vi "MTM2_logEvent_logLevel.vi"(8 "error in (no error)":errorcluster, 11 "logevent_logLevel_Ctl":T1) -> (0 "error out":errorcluster, 2 "function return":i32, 3 "logevent_logLevel_Ctl out":T1)   [LabVIEW 2018, in "SALLV_MTM2.lvlib"]
doc: "int MTM2_shm_logEvent_logLevelLV(MTM2_logevent_logLevelLV *logevent_logLevel_Ctl );"
uses:
  SALLV_MTM2.lvlib
  DataTypes/logevent_logLevel.ctl
  SALLV_MTM2.so
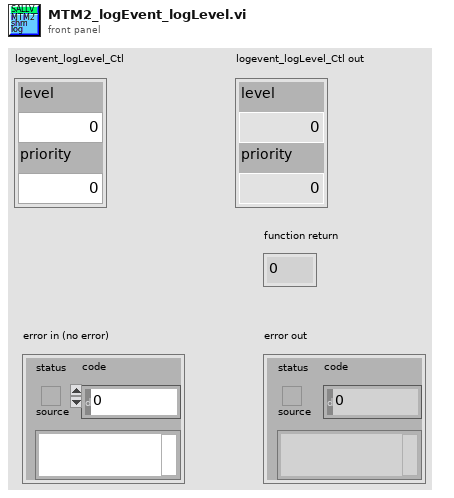
[diagram p1: front panel]
types:
  T1 = typedef "SALLV_MTM2.lvlib/logevent_logLevel.ctl" = cluster{"level":i32, "priority":i32}
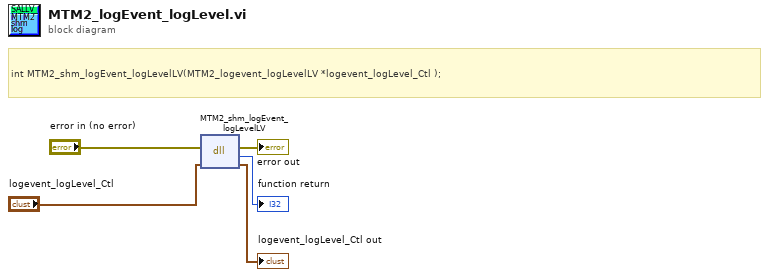
[diagram p0: block diagram]
diagram:
  # "int MTM2_shm_logEvent_logLevelLV(MTM2_logevent_logLevelLV *logevent_logLevel_Ctl );"
  n1 = dll-call lib="home/ttsai/Document/salApiMTM2/SALLV_MTM2/SALLV_MTM2.*" fn="MTM2_shm_logEvent_logLevelLV"(error in="error in (no error)", "logevent_logLevel_Ctl"="logevent_logLevel_Ctl") -> (error out=→"error out":errorcluster, →"function return":i32, "logevent_logLevel_Ctl"=→"logevent_logLevel_Ctl out":T1)  [unwired: 2 in, 1 out]
